vi "FTW-Container-Serialize-JSON.vi"(0 "Container":refnum<class "FTW-Container.lvclass">, 5 "Indent Spaces":i32=4, 11 "error in":errorcluster) -> (4 "Container out":refnum<class "FTW-Container.lvclass">, 6 "Serialized Container":string, 15 "error out":errorcluster)   [LabVIEW 2015, in "FTW-Container.lvclass"]
uses:
  FTW-Container.lvclass
  FTW-Container.lvclass/FTW-Container.ctl
panel:
  # "Inputs"
  # "Outputs"
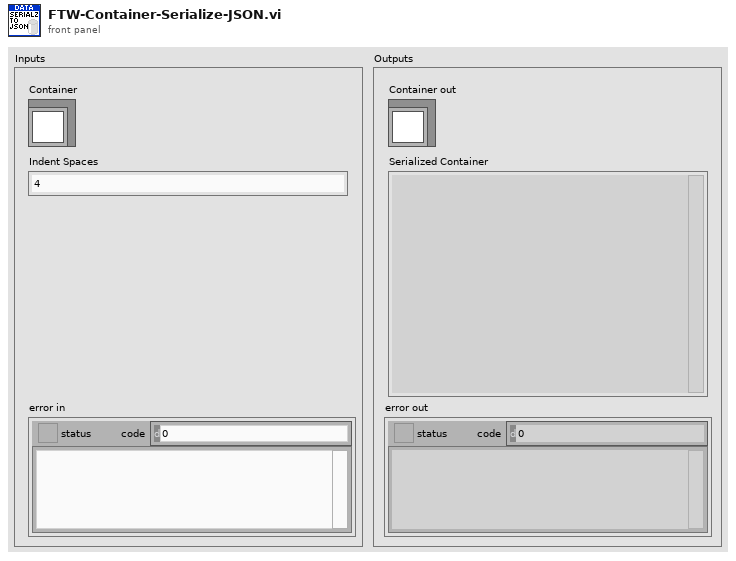
[diagram p1: front panel]
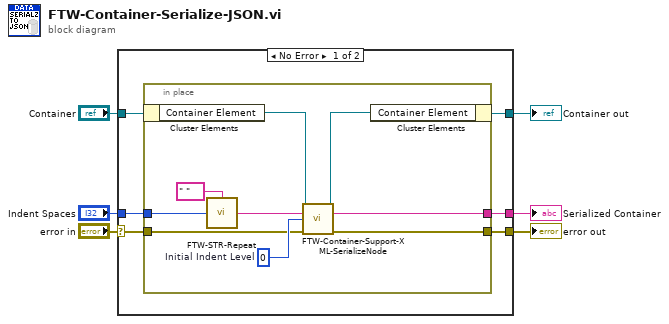
[diagram p0: block diagram]
diagram:
  n1 = case shown="No Error" "error in" {
    selector: "error in" -> [w12 w23]
    tunnel: [w11 w23] -> w6
    tunnel: "Container" -> [w10 w22]
    tunnel: [w9 w22] -> w3
    tunnel: [w8 _] -> w2
    tunnel: "Indent Spaces" -> [w7 _]
    frame No Error {
      n2 = in-place {
        in-place-border: w12 -> [w14]
        in-place-border: [w15] -> w11
        in-place-border: [w19] -> w8
        in-place-border: w7 -> [w21]
        w17 = 0  # Initial Indent Level
        n3 = in-place-cluster #1(w10) -> ("Container Element"=w16:refnum<k20>)
        n4 = call "FTW-STR-Repeat.vi"("Times to Repeat"=w21, "String to Repeat"=" ") -> ("Indented String"=w18:string)
        n5 = call "FTW-Container-Support-XML-SerializeNode.vi"("XML Node"=w16, "Indent Characters"=w18, "Indent Level"=w17, "error in"=w14) -> ("XML Node out"=w13:refnum<k20>, "Serialized Node"=w19:string, "error out"=w15:errorcluster)  [unwired: 9 in]
        n6 = in-place-cluster #1("Container Element"=w13) -> (w9:refnum<class "FTW-Container.lvclass">)
      }
    }
    frame Error {
    }
  }
  "error out" <- w6
  "Serialized Container" <- w2
  "Container out" <- w3
